vi "test-labview-median-function.vi"() -> ()   [LabVIEW 2019]
uses:
  <vilib>/Analysis/NI_AALBase.lvlib
panel:
  out "size(s)":i32
  out "error":i32
  out "Array":dbl[](array[numeric])
  out "MedianValue":dbl
  # "Answer should be 4.5"
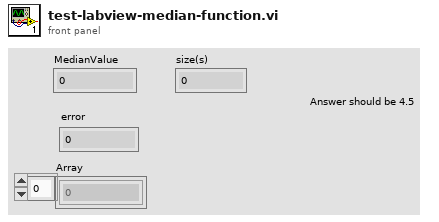
[diagram p1: front panel]
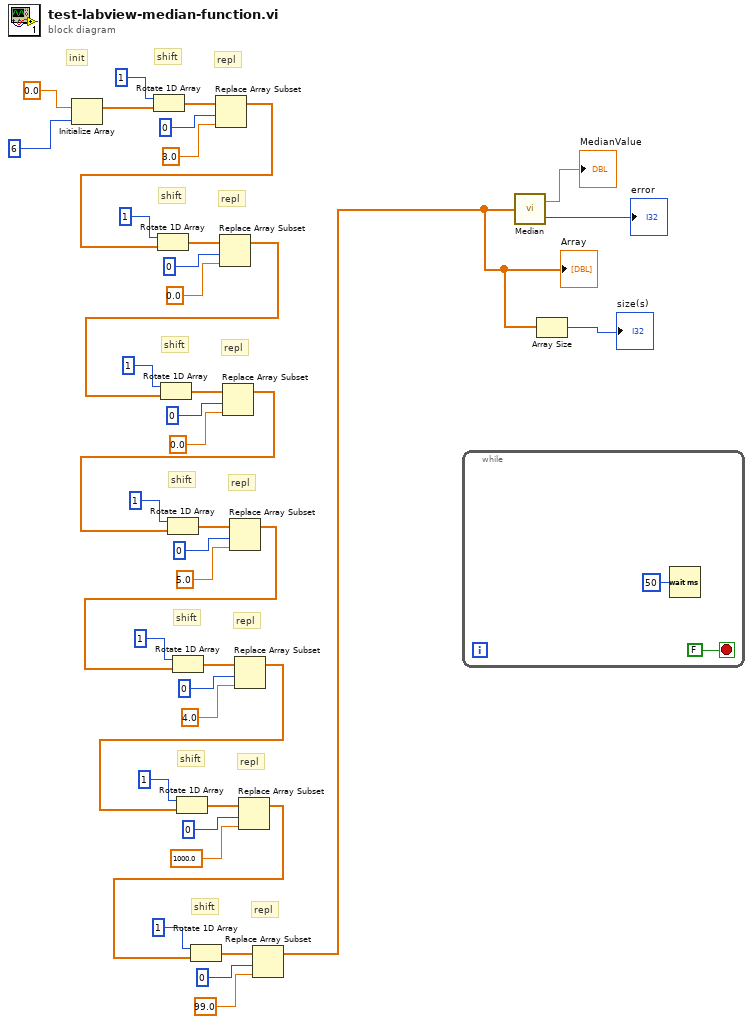
[diagram p0: block diagram]
diagram:
  # "repl"
  # "shift"
  # "repl"
  # "shift"
  # "repl"
  # "shift"
  # "repl"
  # "shift"
  # "repl"
  # "shift"
  # "repl"
  # "shift"
  # "repl"
  # "shift"
  # "init"
  n1 = Initialize Array(0.0 ("element"), 6 ("Samples")) -> (w33:dbl[])
  n2 = Rotate 1D Array(1:w33, 2:1 ("n")) -> (0:w41:dbl[])
  n3 = Replace Array Subset(array=w41, new element=3.0 ("new element/subarray"), index=0) -> (w12:dbl[])
  n4 = Rotate 1D Array(1:w12, 2:1 ("n")) -> (0:w32:dbl[])
  n5 = Replace Array Subset(array=w32, new element=0.0 ("new element/subarray"), index=0) -> (w11:dbl[])
  n6 = Rotate 1D Array(1:w11, 2:1 ("n")) -> (0:w28:dbl[])
  n7 = Replace Array Subset(array=w28, new element=0.0 ("new element/subarray"), index=0) -> (w10:dbl[])
  n8 = Rotate 1D Array(1:w10, 2:1 ("n")) -> (0:w24:dbl[])
  n9 = Replace Array Subset(array=w24, new element=5.0 ("new element/subarray"), index=0) -> (w9:dbl[])
  n10 = Rotate 1D Array(1:w9, 2:1 ("n")) -> (0:w20:dbl[])
  n11 = Replace Array Subset(array=w20, new element=4.0 ("new element/subarray"), index=0) -> (w8:dbl[])
  n12 = Rotate 1D Array(1:w8, 2:1 ("n")) -> (0:w16:dbl[])
  n13 = Replace Array Subset(array=w16, new element=1000.0 ("new element/subarray"), index=0) -> (w3:dbl[])
  n14 = Rotate 1D Array(1:w3, 2:1 ("n")) -> (0:w7:dbl[])
  n15 = Replace Array Subset(array=w7, new element=99.0 ("new element/subarray"), index=0) -> (w2:dbl[])
  "Array" <- w2
  n16 = while {
    stop <- FALSE stop-if-true
    n17 = Wait (ms)(milliseconds to wait=u32 50) -> ()  [unwired: 1 out]
  }
  n18 = call <vilib>:"Median.vi"("X"=w2) -> ("median"=→"MedianValue":dbl, "error"=→"error":i32)
  n19 = Array Size(array=w2) -> (size(s)=→"size(s)":i32)
